vi "F60_Diagnostic.vi"() -> (2 "Edit BSA Setup Out":bool)   [LabVIEW 2016]
uses:
  Globals/LDA_meas_global_1.vi
  Globals/LDA_meas_global_2.vi
panel:
  out "Data 2":dbl[](graph)
  in  "Configuration":string(combo)="0"
  in  "samples":i32=500
  in  "time (s)":sgl=5.0
  in  "Edit BSA Setup":bool
  out "Data":dbl[](graph)
  in  "Start ACQ":bool
  in  "stop":bool
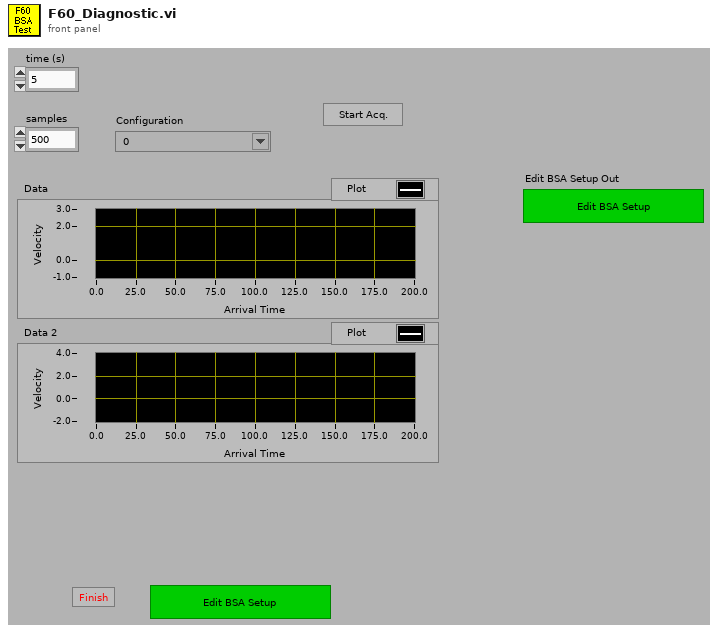
[diagram p1: front panel]
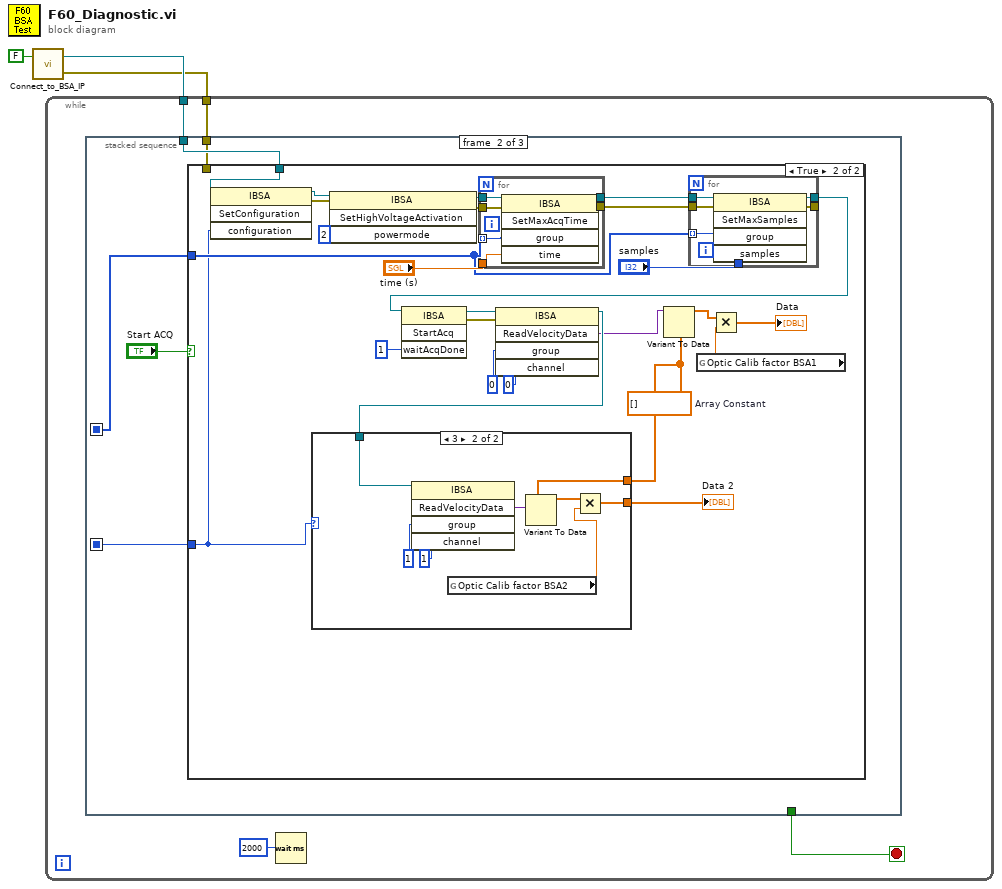
[diagram p0: block diagram]
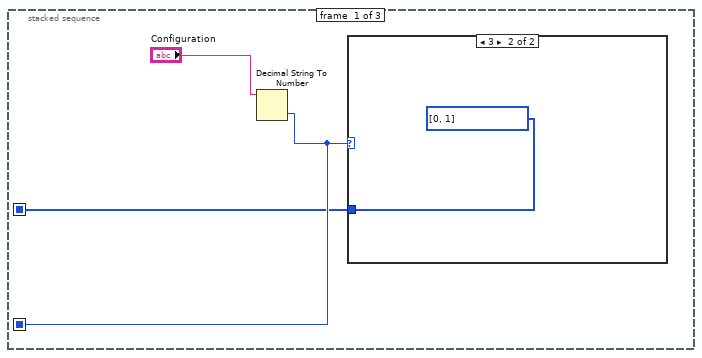
[diagram p2: hidden frame]
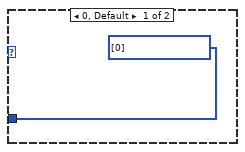
[diagram p3: hidden frame]
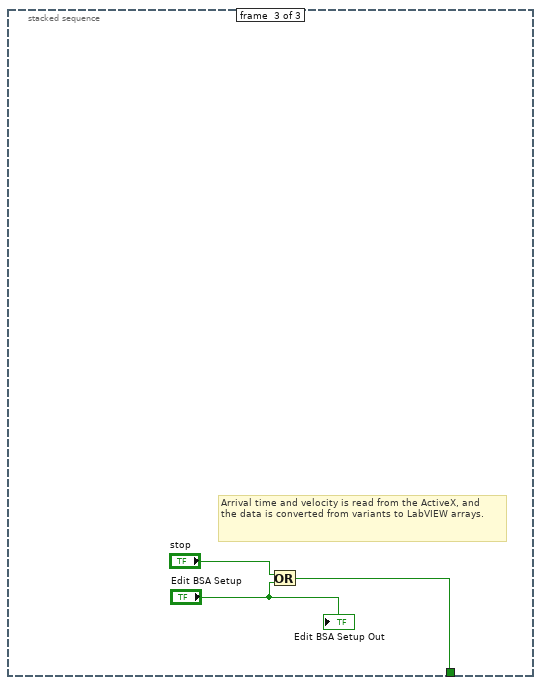
[diagram p6: hidden frame]
diagram:
  n1 = call "Connect_to_BSA_IP.vi"("Force Reconnect"=FALSE) -> ("error out"=w2:errorcluster, "BSA"=w3:refnum<k7>)  [unwired: 1 out]
  n2 = while {
    tunnel: w3 -> [w7]
    tunnel: w2 -> [w6]
    stop <- w5 stop-if-true
    n3 = stacked-sequence {
      seq-local: [w9 _ _] -> [_ w13 _]
      seq-local: [w8 _ _] -> [_ w14 _]
      tunnel: w7 -> [_ w16 _]
      tunnel: w6 -> [_ w15 _]
      tunnel: [_ _ w66] -> w5
      frame #0 {
        n4 = Decimal String To Number(string="Configuration") -> (number=w9:i32)  [unwired: 3 out]
        n5 = case shown="3" w9 {
          tunnel: [i32[] [0] i32[] [0, 1]] -> w8
          frame 0, Default {
          }
          frame 3 {
          }
        }
      }
      frame #1 {
        n6 = case shown="True" "Start ACQ" {
          tunnel: w16 -> [_ w22]
          tunnel: w15 -> [_ _]
          tunnel: w14 -> [_ w24]
          tunnel: w13 -> [_ w21]
          frame False {
          }
          frame True {
            w27 = dbl[] []  # Array Constant
            n7 = invoke class="IBSA" method="SetConfiguration"(reference=w22, "configuration"=w21) -> (reference out=w19:refnum<k7>, error out=w18:errorcluster)  [unwired: 2 in, 2 out]
            n8 = invoke class="IBSA" method="SetHighVoltageActivation"(reference=w19, error in=w18, "powermode"=2) -> (reference out=w41:refnum<k7>, error out=w42:errorcluster)  [unwired: 1 in, 2 out]
            n9 = for {
              tunnel: w42 -> [w54]
              tunnel: w41 -> [w53]
              tunnel: "time (s)" -> [w52]
              tunnel: [w51] -> w39
              tunnel: [w50] -> w38
              tunnel: w24 -> [w49] mode=indexing
              n10 = invoke class="IBSA" method="SetMaxAcqTime"(reference=w53, error in=w54, "group"=w49, "time"=w52) -> (reference out=w51:refnum<k7>, error out=w50:errorcluster)  [unwired: 1 in, 3 out]
            }
            n11 = for {
              tunnel: w24 -> [w48] mode=indexing
              tunnel: w39 -> [w47]
              tunnel: w38 -> [w46]
              tunnel: "samples" -> [w45]
              tunnel: [w44] -> w20
              tunnel: [w43] -> _
              n12 = invoke class="IBSA" method="SetMaxSamples"(reference=w47, error in=w46, "group"=w48, "samples"=w45) -> (reference out=w44:refnum<k7>, error out=w43:errorcluster)  [unwired: 1 in, 3 out]
            }
            n13 = invoke class="IBSA" method="StartAcq"(reference=w20, "waitAcqDone"=1) -> (reference out=w32:refnum<k7>, error out=w33:errorcluster)  [unwired: 2 in, 2 out]
            n14 = invoke class="IBSA" method="ReadVelocityData"(reference=w32, error in=w33, "group"=0, "channel"=0 ("ich")) -> (reference out=w28:refnum<k7>, "ReadVelocityData"=w25:variant)  [unwired: 1 in, 3 out]
            n15 = case shown="3" w21 {
              tunnel: w28 -> [_ w61]
              tunnel: w27 -> [w55 w60]
              tunnel: [w55 w57] -> w26
              frame 0, Default {
              }
              frame 3 {
                n16 = invoke class="IBSA" method="ReadVelocityData"(reference=w61, "group"=1, "channel"=1 ("ich")) -> ("ReadVelocityData"=w59:variant)  [unwired: 2 in, 4 out]
                n17 = global read "LDA_meas_global_2.vi" "Optic Calib factor BSA2"() -> (w56:dbl)
                n18 = Variant To Data(type=w60, Variant=w59) -> (data=w58:dbl[])  [unwired: 1 in, 1 out]
                n19 = Multiply(x=w58, y=w56) -> (x*y=w57:dbl[])
              }
            }
            "Data 2" <- w26
            n20 = Variant To Data(type=w27, Variant=w25) -> (data=w30:dbl[])  [unwired: 1 in, 1 out]
            n21 = global read "LDA_meas_global_1.vi" "Optic Calib factor BSA1"() -> (w31:dbl)
            n22 = Multiply(x=w30, y=w31) -> (x*y=→"Data":dbl[])
          }
        }
      }
      frame #2 {
        # "Arrival time and velocity is read from the ActiveX, and \nthe data is converted from variants to LabVIEW arrays."
        n23 = Or(x="stop", y="Edit BSA Setup") -> (x .or. y?=w66:bool)
        "Edit BSA Setup Out" <- "Edit BSA Setup"
      }
    }
    n24 = Wait (ms)(milliseconds to wait=u32 2000) -> ()  [unwired: 1 out]
  }
